vi "E03_EstructurFor.vi"() -> ()   [LabVIEW 2026]
panel:
  out "Waveform Chart":dbl(graph)
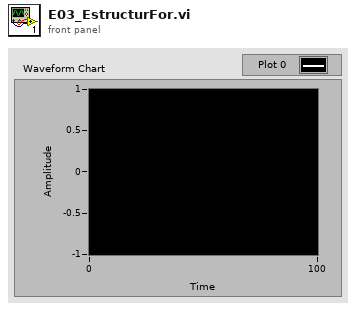
[diagram p1: front panel]
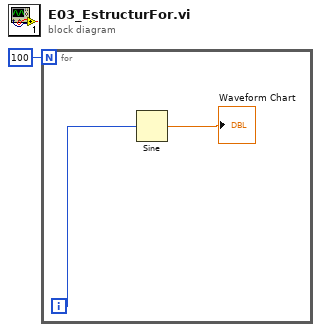
[diagram p0: block diagram]
diagram:
  n1 = for {
    N: 100 -> [_]
    i -> [w2]
    n2 = Sine(x=w2) -> (sin(x)=→"Waveform Chart":dbl)
  }
